vi "Check executables admin priviledges.vi"() -> (0 "error out":errorcluster, 3 "Exe not run as an administrator":bool)   [LabVIEW 2020]
uses:
  Typedefs/Which path.ctl
  <vilib>/Utility/config.llb/Read Key (Boolean).vi
  <vilib>/Utility/config.llb/Write Key (Boolean).vi
  <vilib>/Utility/config.llb/NI_LVConfig.lvlib
panel:
  out "Application:Kind":T1(ring)
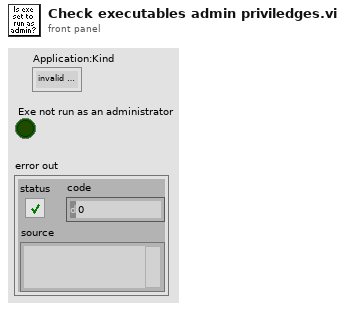
[diagram p1: front panel]
types:
  T1 = enum32{"invalid app kind", "Development System", "Run Time System", "Student Edition", "Embedded LabVIEW", "Evaluation", "Custom"}
  T2 = typedef "Which path.ctl" = enum16{"Configuration Files", "Calibration Files", "Images", "Setup.ini", "Loaded User profile.ini", "User's-Previous session.ini", "New user profile.ini", "Selected User profile.ini", "User profiles folder", "Power meter scaling.txt", "FOV Cal.ini", "Calibration.ini"}
  T3 = typedef "NI_LVConfig.lvlib/Config Data RefNum.ctl" = refnum<k1>
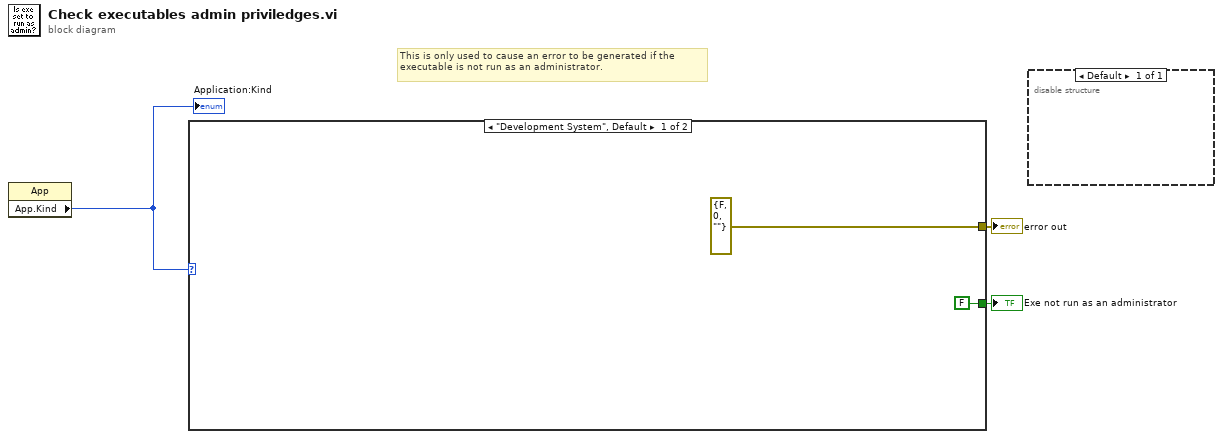
[diagram p0: block diagram]
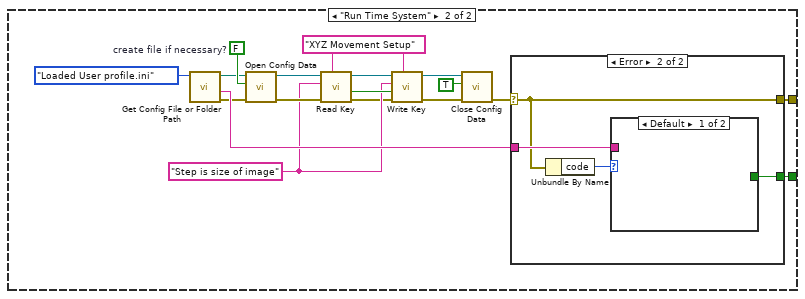
[diagram p2: hidden frame]
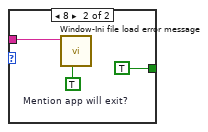
[diagram p4: hidden frame]
diagram:
  # "This is only used to cause an error to be generated if the executable is not run as an administrator."
  n1 = property class="App"() -> ("App.Kind"=w1:T1)  [unwired: 2 in, 2 out]
  "Application:Kind" <- w1
  n2 = case shown="\"Development System\", Default" w1 {
    tunnel: [FALSE w7] -> w3
    tunnel: [errorcluster {"status"=FALSE, "code"=0, "source"=""} ("error IO") w6] -> w2
    frame "Development System", Default {
    }
    frame "Run Time System" {
      w9 = "Step is size of image" ("key")
      w10 = "XYZ Movement Setup" ("section")
      w22 = FALSE  # create file if necessary?
      n3 = call "Get Config File or Folder Path.vi"("Which file or folder?"=Which_path."Loaded User profile.ini" ("Which path?")) -> ("Error Out"=w18:errorcluster, "File/Folder name string"=w19:string, "File Path"=w17:path)  [unwired: 8 in]
      n4 = call <vilib>:"Open Config Data.vi"("error in (no error)"=w18, "create file if necessary (T)"=w22, "configuration file path"=w17) -> ("error out"=w16:errorcluster, "refnum"=w13:T3)  [unwired: 6 in, 1 out]
      n5 = call-poly <vilib>:"Read Key.vi"("section"=w10, "error in (no error)"=w16, "key"=w9, "refnum"=w13) -> ("error out"=w8:errorcluster, "value"=w11:bool, "refnum out"=w14:T3)  [unwired: 4 in, 1 out]
      n6 = call-poly <vilib>:"Write Key.vi"("section"=w10, "error in (no error)"=w8, "value"=w11, "key"=w9, "refnum"=w14) -> ("error out"=w15:errorcluster, "refnum out"=w12:T3)  [unwired: 4 in, 1 out]
      n7 = call <vilib>:"Close Config Data.vi"("error in (no error)"=w15, "write file if changed (T)"=TRUE ("write configuration file? (F)"), "refnum"=w12) -> ("error out"=w23:errorcluster)  [unwired: 7 in, 1 out]
      n8 = case shown="Error" w23 {
        selector: w23 -> [w24 w27]
        tunnel: w19 -> [_ w28]
        tunnel: [w24 w27] -> w6
        tunnel: [_ w25] -> w7
        frame No Error {
        }
        frame Error {
          n9 = Unbundle By Name(w27) -> ("code"=w26:i32)
          n10 = case shown="Default" w26 {
            tunnel: w28 -> [_ w31]
            tunnel: [_ TRUE] -> w25
            frame Default {
            }
            frame 8 {
              w30 = TRUE  # Mention app will exit?
              n11 = call "Window-Ini file load error message.vi"("Mention app will exit? (F)"=w30, "Message"=w31) -> ()  [unwired: 9 in, 1 out]
            }
          }
        }
      }
    }
  }
  "error out" <- w2
  "Exe not run as an administrator" <- w3
  n12 = disable-structure shown="Default" {
    frame Enabled {
    }
  }
